vi "visionFGV.vi"(8 "Error In":errorcluster, 11 "Function":enum16{"set", "readColor", "close", "readGray"}(ring)) -> (0 "error out":errorcluster, 3 "Image Out fgv":T1(plugin-control))   [LabVIEW 2019]
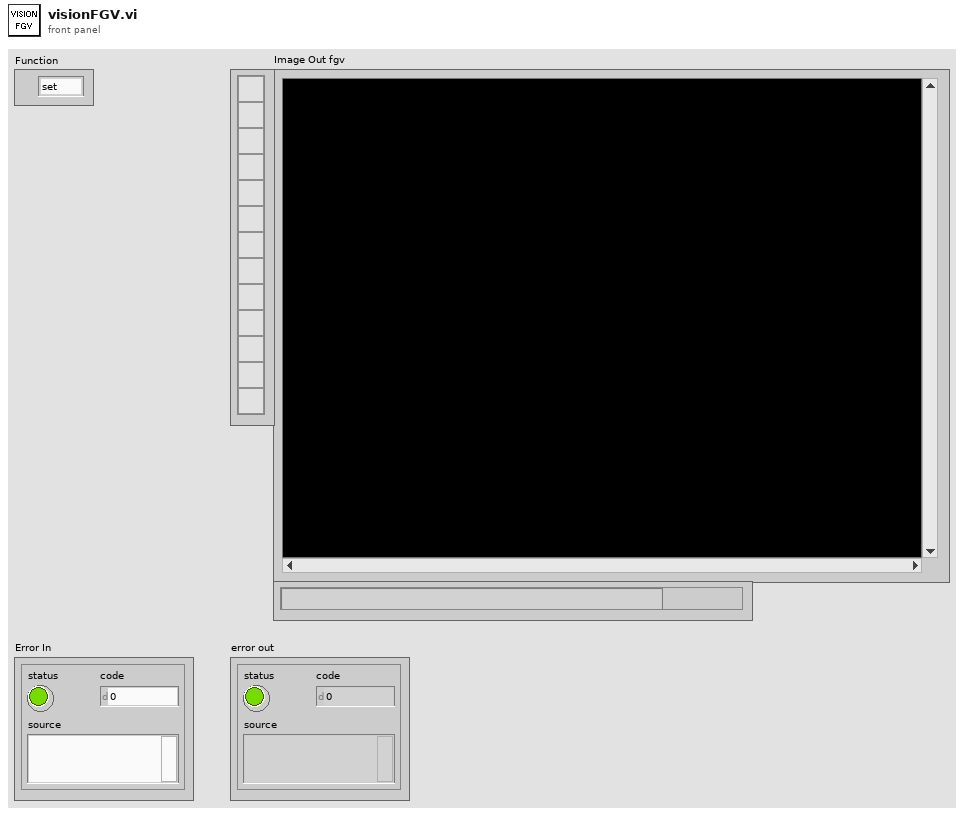
[diagram p1: front panel]
types:
  T1 = typedef "IMAQ Image.ctl" = refnum<image>
  T2 = typedef "Image Type" = u32
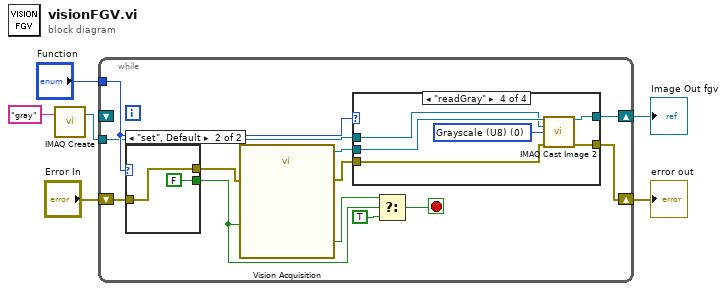
[diagram p0: block diagram]
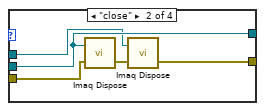
[diagram p3: hidden frame]
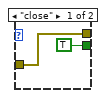
[diagram p5: hidden frame]
diagram:
  n1 = call "IMAQ Create"("Image Name"="gray") -> ("New Image"=w1:T1)  [unwired: 4 in, 1 out]
  n2 = while {
    tunnel: "Function" -> [w15]
    shift-right: [w18] -> w5
    shift-left: "Error In" -> [w17]
    shift-right: [w16] -> w4
    shift-left: _ -> [_]
    tunnel: w1 -> [w7]
    stop <- w14 stop-if-true
    n3 = case shown="\"set\", Default" w15 {
      tunnel: [w35 w36] -> w12
      tunnel: [TRUE ("Stop (F)") FALSE ("Stop (F)")] -> w11
      tunnel: w17 -> [w35 w36]
      frame "close" {
      }
      frame "set", Default {
      }
    }
    n4 = call "Vision Acquisition"("Stop (F)"=w11, "error in"=w12) -> ("Image Out"=w8:T1, "Stopped"=w10:bool, "error out"=w9:errorcluster)  [unwired: 23 in]
    n5 = case shown="\"readGray\"" w15 {
      tunnel: [w20 w21 w26 w29] -> w18
      tunnel: w9 -> [w20 w25 w26 w30]
      tunnel: w8 -> [w19 w24 w27 w33]
      tunnel: [w19 w24 w27 w32] -> w16
      tunnel: w7 -> [_ w22 _ w28]
      frame "readColor" {
      }
      frame "close" {
        n6 = call "Imaq Dispose"("Image"=w24, "error in (no error)"=w25) -> ("error out"=w23:errorcluster)  [unwired: 4 in]
        n7 = call "Imaq Dispose"("Image"=w22, "error in (no error)"=w23) -> ("error out"=w21:errorcluster)  [unwired: 4 in]
      }
      frame Default {
      }
      frame "readGray" {
        w31 = T2 0 items=["Grayscale (U8)", "Grayscale (I16)", "Grayscale (SGL)", "Complex (CSG)", "RGB (U32)", "HSL (U32)", "RGB (U64)", "Grayscale (U16)"] ("Image Type")
        n8 = call "IMAQ Cast Image 2"("Image Src"=w33, "Image Dst"=w28, "Image Type"=w31, "error in (no error)"=w30) -> ("Image Dst Out"=w32:T1, "error out"=w29:errorcluster)  [unwired: 10 in]
      }
    }
    n9 = Select(t=w10, s=w11, f=TRUE) -> (s? t:f=w14:bool)
  }
  "Image Out fgv" <- w4
  "error out" <- w5
